vi "PRL Read Buffer .vi"(10 "Get All Signals":bool, 11 "Get Full Buffer":bool) -> (0 "Digital Signals":bool[][](array[boolean]), 1 "Analog Signals":sgl[][](array[numeric]), 2 "Phasor Signals":csg[][](array[numeric]), 3 "Timestamp":timestamp[](array[timestamp]), 4 "Has Data":bool, 6 "First Buffer Filled":bool)   [LabVIEW 2017, in "PMU Recorder Light.lvlib"]
doc: "Reads the newest data from the PRL Accsess Buffer."
uses:
  PMU Recorder Light.lvlib
panel:
  out "error out":errorcluster
  in  "error in (no error)":errorcluster
  # "INPUT"
  # "INTERMEDIATE"
  # "OUTPUT"
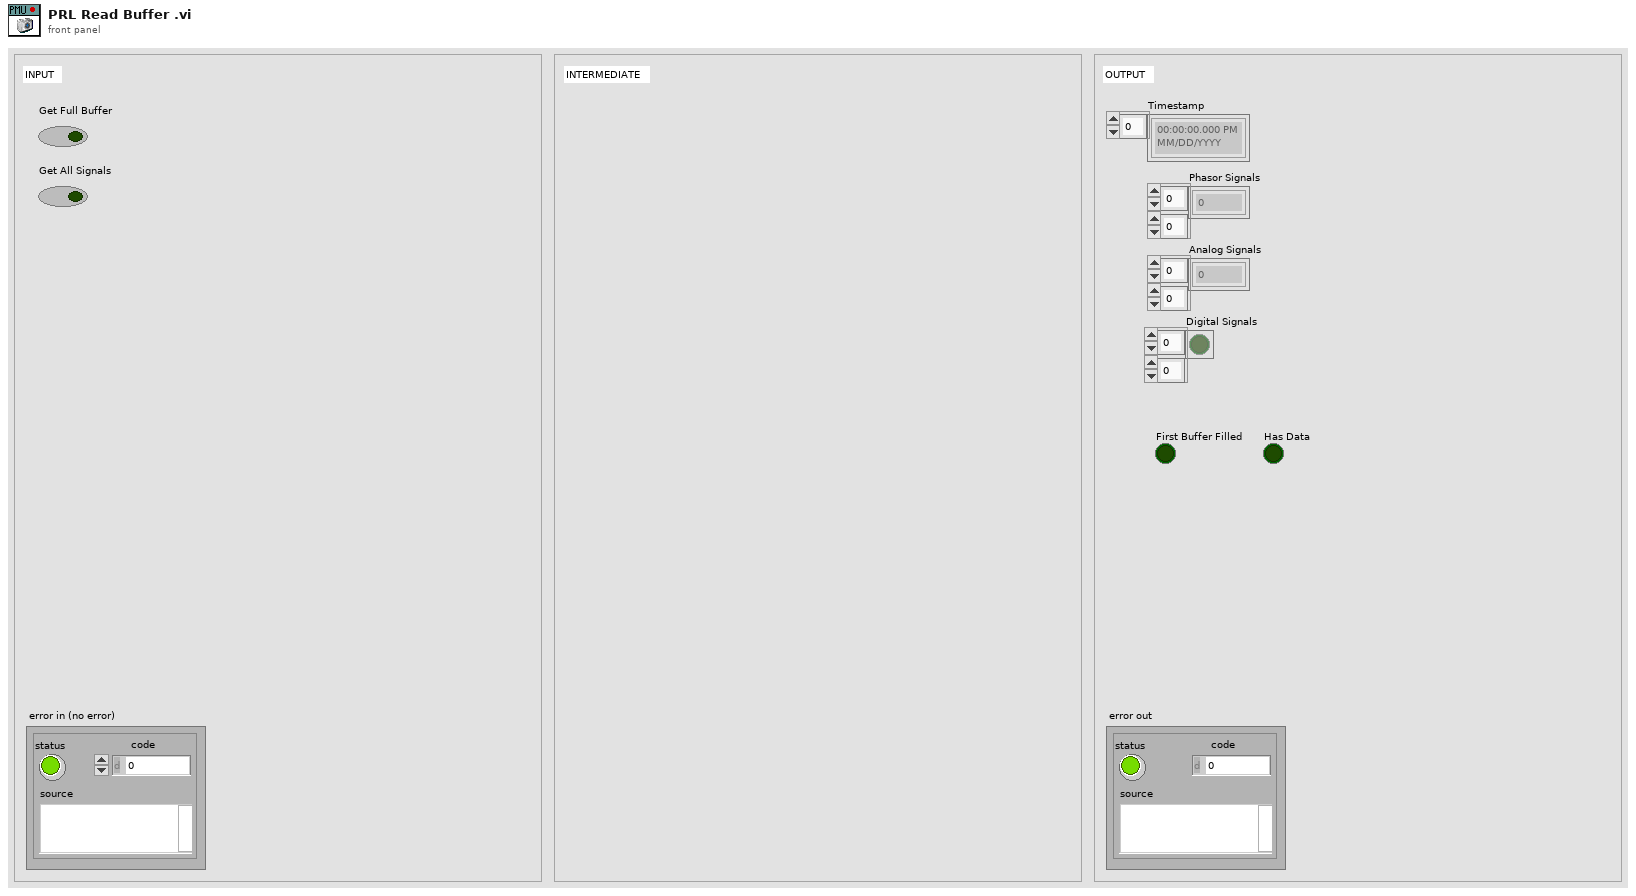
[diagram p1: front panel]
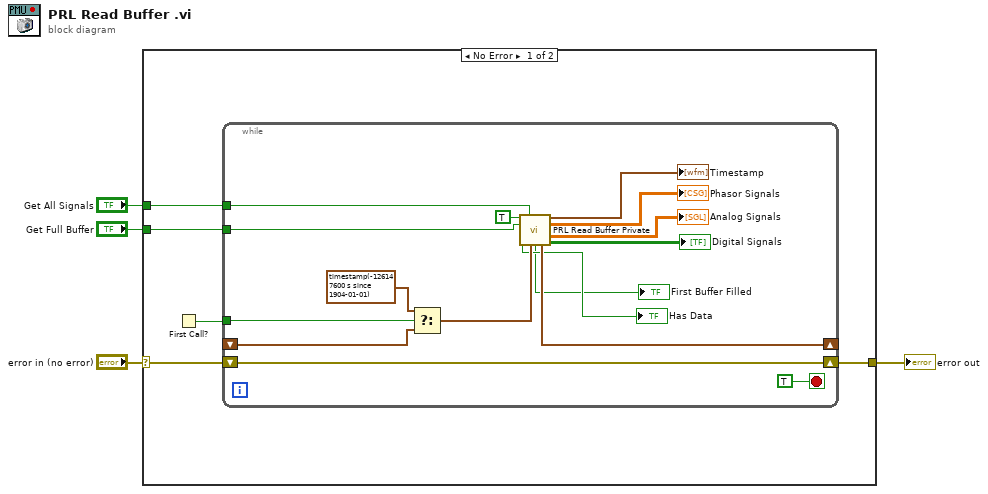
[diagram p0: block diagram]
diagram:
  n1 = case shown="No Error" "error in (no error)" {
    selector: "error in (no error)" -> [w6 w26]
    tunnel: "Get Full Buffer" -> [w8 _]
    tunnel: "Get All Signals" -> [w7 _]
    tunnel: [w5 w26] -> w1
    frame No Error {
      n2 = First Call?() -> (First Call?: T/F=w9:bool)
      n3 = while {
        tunnel: w9 -> [w24]
        shift-right: [w20] -> _
        shift-left: _ -> [w23]
        tunnel: w8 -> [w18]
        tunnel: w7 -> [w17]
        shift-right: [w10] -> w5
        shift-left: w6 -> [w10]
        stop <- TRUE stop-if-true
        n4 = Select(t=timestamp(-126147600 s since 1904-01-01) ("Time  Stamp In"), s=w24, f=w23) -> (s? t:f=w21:timestamp)
        n5 = call "PRL Read Buffer Private.vi"("Read"=TRUE, "Get All Signals"=w17, "Get Full Buffer?"=w18, "Time  Stamp In"=w21) -> ("Timestamp"=→"Timestamp":timestamp[], "Phasor Signals"=→"Phasor Signals":csg[][], "Analog Signals"=→"Analog Signals":sgl[][], "Has Data?"=→"Has Data":bool, "First Buffer Filled"=→"First Buffer Filled":bool, "Time Stamp Out"=w20:timestamp, "Digital Signals"=→"Digital Signals":bool[][])  [unwired: 4 in, 1 out]
      }
    }
    frame Error {
    }
  }
  "error out" <- w1
